vi "Test Glyph on Case Correct on Start Test.vi"(8 "error in (no error)":errorcluster, 11 "Result Model Tests in":refnum<class "Result Model Test Enumeration.lvclass">) -> (0 "error out":errorcluster, 3 "Result Model Tests out":refnum<class "Result Model Test Enumeration.lvclass">)   [LabVIEW 2020, in "Result Model Test Enumeration.lvclass"]
uses:
  Result Model Test Enumeration.lvclass
  source/User Interface/Result Model/Result Model.lvclass
  206db1ee-aa99-40b9-8881-171f2a77c34b.vi
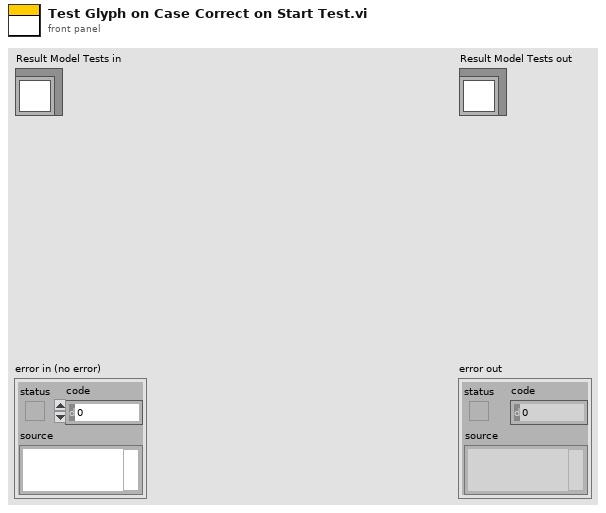
[diagram p1: front panel]
types:
  T1 = cluster{"Left Cell String":string, "Child Text":string[], "Child Tag":string, "Item Indent":i32, "Child Only?":bool, "Glyph Index":i32}[]
  T2 = cluster{"Left Cell String":string, "Child Text":string[], "Child Tag":string, "Item Indent":i32, "Child Only?":bool, "Glyph Index":i32}
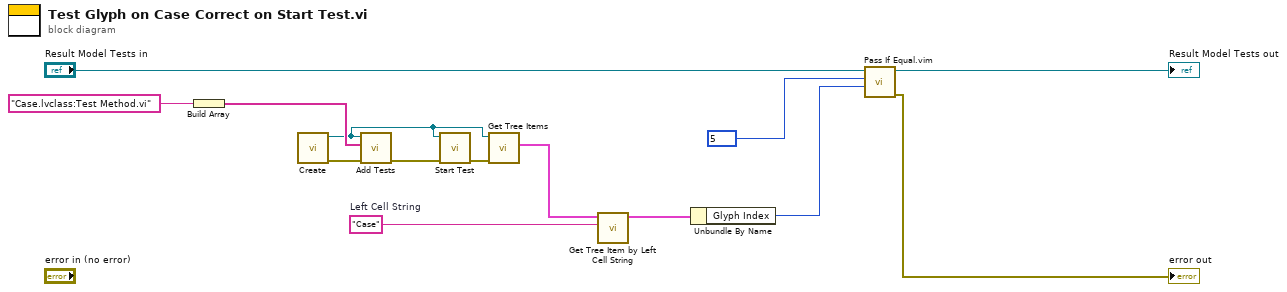
[diagram p0: block diagram]
diagram:
  w6 = "Case"  # Left Cell String
  n1 = Build Array("Case.lvclass:Test Method.vi" ("String")) -> (w9:string[])
  n2 = call "Create.vi"() -> ("error out"=w4:errorcluster, "Result Model out"=w1:refnum<class "Result Model.lvclass">)  [unwired: 10 in]
  n3 = call "Add Tests.vi"("error in (no error)"=w4, "Tests"=w9, "Result Model by Reference In"=w1) -> ("error out"=w3:errorcluster)  [unwired: 8 in]
  n4 = call "Start Test.vi"("error in (no error)"=w3, "Result Model by Reference In"=w1) -> ("error out"=w2:errorcluster)  [unwired: 9 in]
  n5 = call "Get Tree Items.vi"("error in (no error)"=w2, "Result Model by Reference In"=w1) -> ("Tree Items"=w13:T1)  [unwired: 8 in, 1 out]
  n6 = call "Get Tree Item by Left Cell String.vi"("Left Cell String"=w6, "Tree Items"=w13) -> ("Item"=w11:T2)  [unwired: 9 in]
  n7 = Unbundle By Name(w11) -> ("Glyph Index"=w10:i32)
  n8 = call "Pass If Equal.vim"("Actual"=w10, "Expected"=5 ("Listbox Symbol Ring Constant"), "LUnit Test Case In"="Result Model Tests in") -> ("error out"=→"error out":errorcluster, "LUnit Test Case Out"=→"Result Model Tests out":refnum<class "Result Model Test Enumeration.lvclass">)  [unwired: 7 in]
